vi "NHMFL User Bank Server.vi"() -> ()   [LabVIEW 2015]
uses:
  Library/Shot data.ctl
  Library/OPC Adresses.ctl
panel:
  out "remote port":u16
  out "remote address":string
  out "Formated shot data":string
  out "Stop TCP server":bool
  in  "OPC adressess":T1={"Data Received  URL"="opc:\\cyberlogic.opcserverDA\\UB.DataReceived", "Data Ready URL"="opc:\\cyberlogic.opcserverDA\\UB.DataReady", "Message URL"="opc:\\cyberlogic.opcserverDA\\UB.MagHistString"}
  in  "Test":bool
  in  "Log file folder":path=path "C:/Data"
  out "error out":errorcluster
  out "Last shot data":T2
  in  "stop":bool
  out "Data Ready":bool
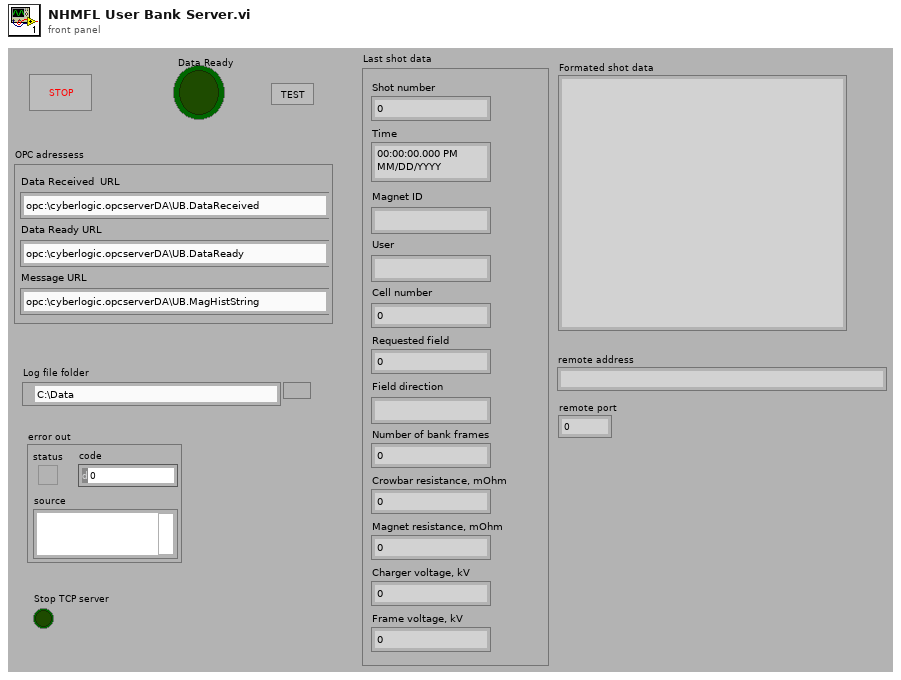
[diagram p1: front panel]
types:
  T1 = typedef "OPC Adresses.ctl" = cluster{"Data Received  URL":string, "Data Ready URL":string, "Message URL":string}
  T2 = typedef "Shot data.ctl" = cluster{"Shot number":i32, "Time":timestamp, "Magnet ID":string, "User":string, "Cell number":i32, "Requested field":dbl, "Field direction":string, "Number of bank frames":i32, "Crowbar resistance, mOhm":dbl, "Magnet resistance, mOhm":dbl, "Charger voltage, kV":dbl, "Frame voltage, kV":dbl}
  T3 = typedef "OPC connections.ctl" = cluster{"Data received":refnum<k13>, "Data Ready":refnum<k13>, "Message":refnum<k13>}
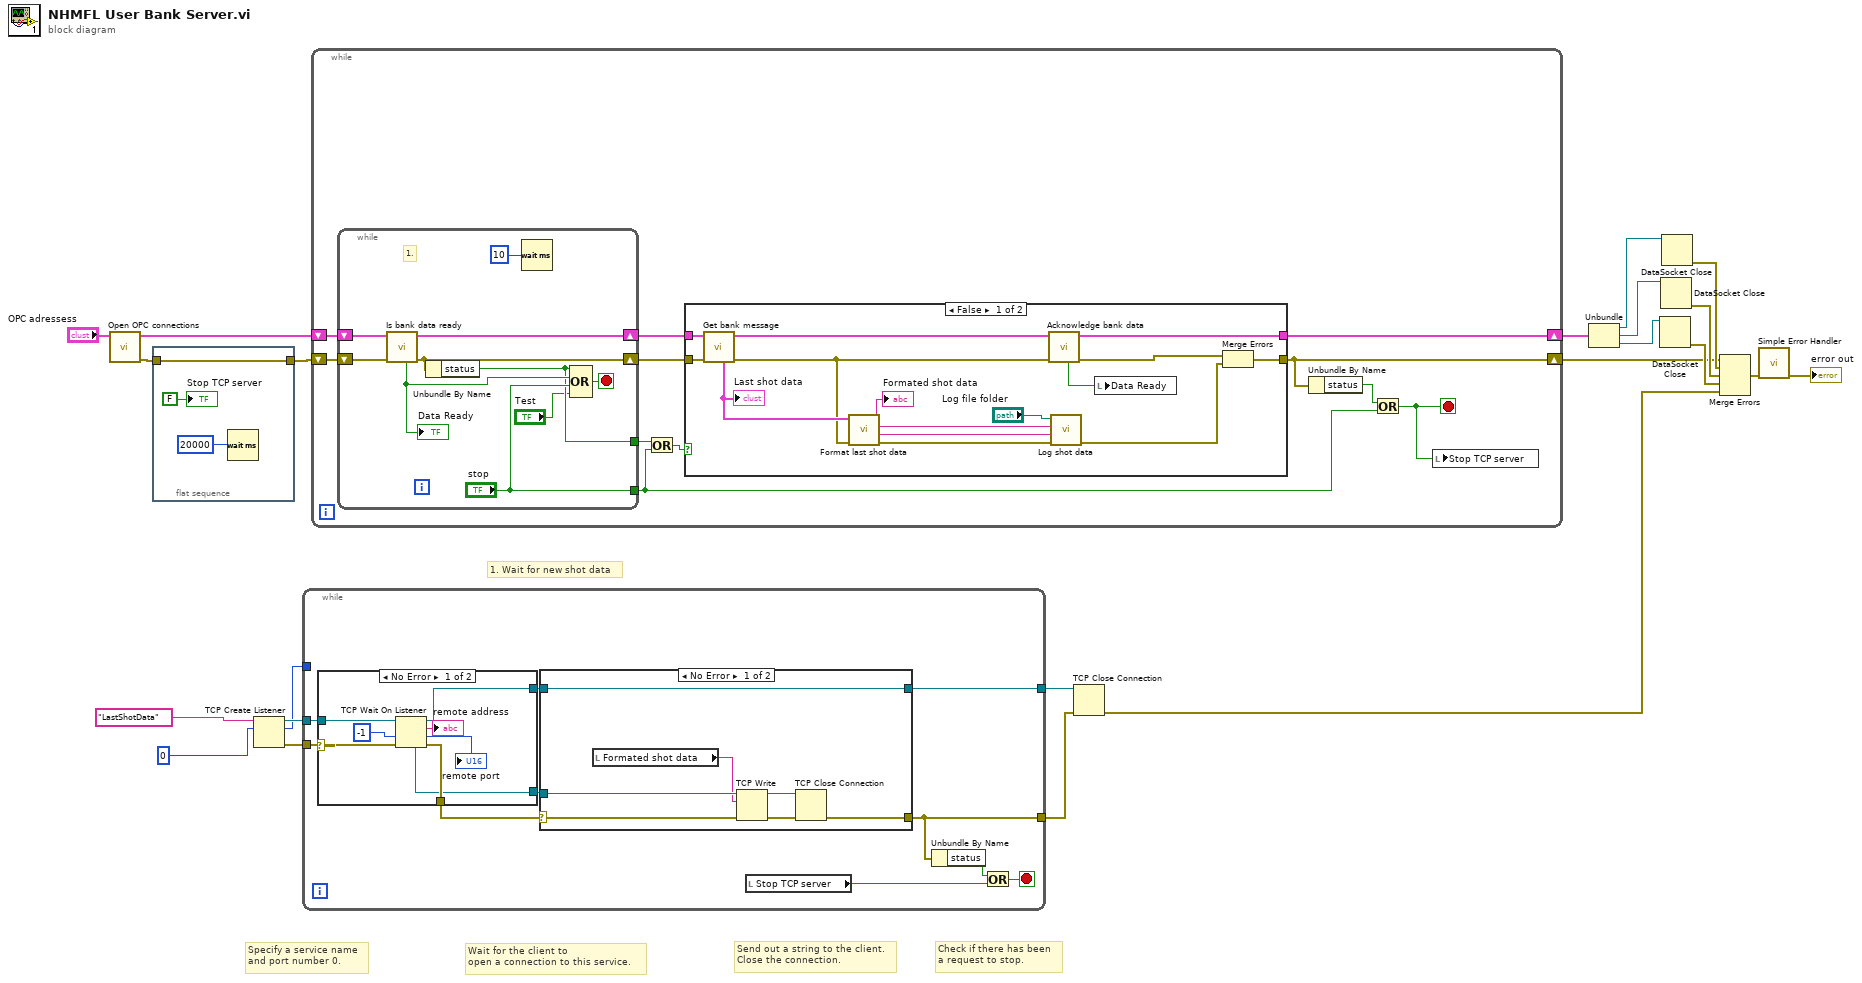
[diagram p0: block diagram]
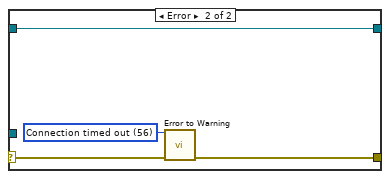
[diagram p2: hidden frame]
diagram:
  # "Check if there has been\na request to stop."
  # "Wait for the client to\nopen a connection to this service."
  # "Send out a string to the client.\nClose the connection."
  # "Specify a service name\nand port number 0."
  # "1. Wait for new shot data"
  n1 = call "Open OPC connections.vi"("OPC adressess"="OPC adressess") -> ("error IO"=w21:errorcluster, "OPC connections"=w19:T3)  [unwired: 9 in]
  n2 = flat-sequence {
    tunnel: [w25] -> w22
    tunnel: w21 -> [w25]
    frame #0 {
      n3 = Wait (ms)(milliseconds to wait=u32 20000) -> ()  [unwired: 1 out]
      "Stop TCP server" <- FALSE ("Stop TCP server")
    }
  }
  n4 = TCP Create Listener(10:u16 0, 11:"LastShotData") -> (0:w5:errorcluster, 2:w4:u16, 3:w6:refnum<k5>)  [unwired: 3 in]
  n5 = while {
    tunnel: w6 -> [w35]
    tunnel: w5 -> [w33]
    tunnel: [w27] -> w2
    tunnel: w4 -> [_]
    tunnel: [w31] -> w3
    stop <- w29 stop-if-true
    n6 = case shown="No Error" w33 {
      selector: w33 -> [w53 w55]
      tunnel: w35 -> [w54 _]
      tunnel: [w52 w55] -> w30
      tunnel: [w51 _] -> w34
      tunnel: [w49 _] -> w32
      frame No Error {
        n7 = TCP Wait On Listener(8:w53, 9:-1, 11:w54) -> (0:w52:errorcluster, 1:→"remote port":u16, 2:→"remote address":string, 3:w49:refnum<k5>, 4:w51:refnum<k5>)  [unwired: 1 in]
      }
      frame Error {
      }
    }
    n8 = case shown="No Error" w30 {
      selector: w30 -> [w38 w44]
      tunnel: [w41 w43] -> w27
      tunnel: w34 -> [w42 _]
      tunnel: [w37 w46] -> w31
      tunnel: w32 -> [w37 w46]
      frame No Error {
        n9 = local read "Formated shot data"() -> (w36:string)
        n10 = TCP Write(connection ID=w42, data in=w36, error in (no error)=w38) -> (connection ID out=w39:refnum<k5>, error out=w40:errorcluster)  [unwired: 1 in, 1 out]
        n11 = TCP Close Connection(connection ID=w39, error in (no error)=w40) -> (error out=w41:errorcluster)  [unwired: 1 in, 1 out]
      }
      frame Error {
        w45 = 56 items=["No Error", "Argument Error", "Memory Full", "Out of Zone", "End of File", "File Already Open", "Generic File IO Error", "File Not Found", "File Permission Error", "Disk Full", "Duplicate Path", "Too Many Files Open", "Not Enabled", "Resource File Not Found", "Cannot Add Resource", "Resource Not Found", "Image Not Found", "Image Memory Error", "Pen Does Not Exist", "Config Bad Type", "Config Token Not Found", "Config Parse Error", "Config Memory Error", "Bad External Code Format", "Bad External Code Offset", "External Code Not Present", "Null Window", "Destroy Window Mixup", "Null Menu", "Print Aborted", "Bad Print Record", "Print Driver Error", "Windows Error During Print", "Memory Error During Print", "Print Dialog Error", "Generic Print Error", "Invalid Device Refnum", "Device Not Found", "Device Parameter Error", "Device Unit Error", "Can't Open Device", "Device Call Aborted", "Generic Error", "Cancelled By User", "Object ID Too Low", "Object ID Too High", "Object Not In Heap", "Unknown Heap", "Bad DefProc ID", "DefProc Not In Table", "Message Out Of Range", "Null Method", "Unknown Message", "Manager Call Not Supported", "Bad address", "Connection In progress", "Connection timed out", "Connection is already in progress", "Network attribute not supported", "Network error", "Address in use", "System out of memory", "Connection aborted", "Connection refused", "Connection is not connected", "Connection is already connected", "Connection closed", "Initialize error (interapplication manager)", "Bad occurrence", "Wait on unbound occurrence handler", "Occurrence queue overflow", "Bad path", "Semaphore not signaled", "Unrecognized type (interapplication manager)"] ("1st Error to Convert")
        n12 = call <vilib>:"Error to Warning.vi"("1st Error to Convert"=w45, "error in"=w44) -> ("warning out"=w43:errorcluster)  [unwired: 13 in]
      }
    }
    n13 = local read "Stop TCP server"() -> (w26:bool)
    n14 = Unbundle By Name(w27) -> ("status"=w28:bool)
    n15 = Or(x=w28, y=w26) -> (x .or. y?=w29:bool)
  }
  n16 = while {
    shift-right: [w64] -> w9
    shift-left: w22 -> [w66]
    shift-right: [w60] -> w18
    shift-left: w19 -> [w62]
    stop <- w63 stop-if-true
    n17 = while {
      tunnel: ["stop"] -> w57
      shift-right: [w91] -> w65
      shift-left: w66 -> [w92]
      shift-right: [w89] -> w61
      shift-left: w62 -> [w90]
      tunnel: [w86] -> w58
      stop <- w85 stop-if-true
      # "1."
      n18 = call "Is bank data ready.vi"("error IO"=w92, "OPC connections"=w90) -> ("error out"=w91:errorcluster, "OPC connections out"=w89:T3, "Data ready"=w87:bool)  [unwired: 7 in]
      "Data Ready" <- w87
      n19 = Unbundle By Name(w91) -> ("status"=w86:bool)
      n20 = Wait (ms)(milliseconds to wait=u32 10) -> ()  [unwired: 1 out]
      n21 = Compound Arithmetic op=OR(w86, w87, "stop", "Test") -> (w85:bool)
    }
    n22 = Or(x=w58, y=w57) -> (x .or. y?=w59:bool)
    n23 = case shown="False" w59 {
      tunnel: w65 -> [w81 w83]
      tunnel: [w79 w83] -> w64
      tunnel: w61 -> [w76 w82]
      tunnel: [w74 w82] -> w60
      frame False {
        n24 = call "Get bank message.vi"("error IO"=w81, "OPC connections"=w76) -> ("error out"=w72:errorcluster, "OPC connections out"=w75:T3, "Shot data"=w73:T2)  [unwired: 4 in, 3 out]
        "Last shot data" <- w73
        n25 = call "Format last shot data.vi"("error in (no error)"=w72, "Shot data"=w73) -> ("error out"=w71:errorcluster, "Spreadsheet header string"=w69:string, "Spreadsheet shot string"=w70:string, "Formated shot data"=→"Formated shot data":string)  [unwired: 5 in, 1 out]
        n26 = call "Acknowledge bank data.vi"("error in"=w72, "OPC connections"=w75) -> ("error out"=w80:errorcluster, "OPC connections out"=w74:T3, "Data ready"=w68:bool)  [unwired: 7 in]
        n27 = call "Log shot data.vi"("error in (no error)"=w71, "Spreadsheet header string"=w69, "Spreadsheet shot string"=w70, "Log file folder"="Log file folder") -> ("error out"=w77:errorcluster)  [unwired: 6 in, 1 out]
        n28 = local write "Data Ready"(w68) -> ()
        n29 = Merge Errors(w80, w77) -> (w79:errorcluster)
      }
      frame True {
      }
    }
    n30 = Unbundle By Name(w64) -> ("status"=w56:bool)
    n31 = Or(x=w56, y=w57) -> (x .or. y?=w63:bool)
    n32 = local write "Stop TCP server"(w63) -> ()
  }
  n33 = TCP Close Connection(connection ID=w3, error in (no error)=w2) -> (error out=w1:errorcluster)  [unwired: 1 in, 1 out]
  n34 = Unbundle(w18) -> ("Data received"=w17:refnum<k13>, "Data Ready"=w16:refnum<k13>, "Message"=w15:refnum<k13>)
  n35 = DataSocket Close(11:w15) -> (0:w12:errorcluster)  [unwired: 2 in, 1 out]
  n36 = DataSocket Close(11:w16) -> (0:w11:errorcluster)  [unwired: 2 in, 1 out]
  n37 = DataSocket Close(11:w17) -> (0:w10:errorcluster)  [unwired: 2 in, 1 out]
  n38 = Merge Errors(w9, w10, w11, w12, w1) -> (w13:errorcluster)
  n39 = call <vilib>:"Simple Error Handler.vi"("error in (no error)"=w13) -> ("error out"=→"error out":errorcluster)  [unwired: 4 in, 4 out]
